vi "2_1_SerieFibonacci.vi"() -> ()   [LabVIEW 2020]
panel:
  out "numero":i32
  out "Serie":dbl[](array[numeric])
  in  "Cant elementos":i32
  out "x*y 2":i32
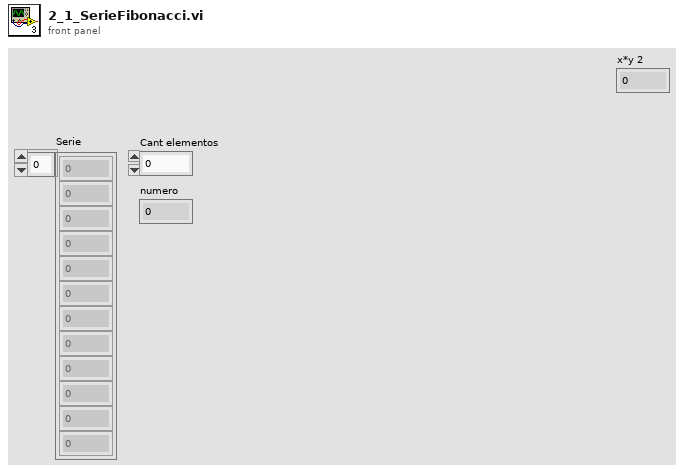
[diagram p1: front panel]
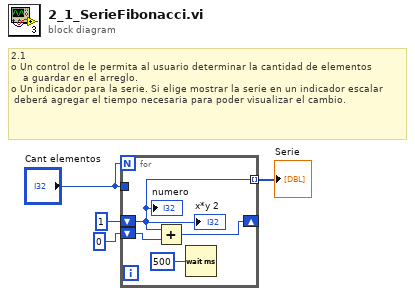
[diagram p0: block diagram]
diagram:
  # "2.1 \no\tUn control de le permita al usuario determinar la cantidad de elementos \n    a guardar en el arreglo.\no\tUn indicador para la serie. Si elige mostrar la serie en un indicador escalar\n deberá agregar el tiempo necesaria para poder visualizar el cambio."
  n1 = for {
    N: "Cant elementos" -> [_]
    shift-right: [w7] -> _
    shift-left: 1 -> [w5]
    shift-left: 0 -> [w8]
    tunnel: "Cant elementos" -> [_]
    tunnel: [w5] -> w1 mode=indexing
    n2 = Add(x=w5, y=w8) -> (x+y=w7:i32)
    n3 = Wait (ms)(milliseconds to wait=500) -> ()  [unwired: 1 out]
    "x*y 2" <- w5
    "numero" <- w5
  }
  "Serie" <- w1
